vi "find_InstrumentObject_by_Name.vi"(10 "Instrument Name":string, 11 "InstrumentObjects":refnum<class "instrument.lvclass">[](array[class])) -> (0 "found?":bool, 1 "index of found":i32, 2 "found InstrObject out":refnum<class "instrument.lvclass">, 3 "InstrumentObjects out":refnum<class "instrument.lvclass">[](array[class]))   [LabVIEW 2017]
doc: "Find the correct IntrumentObject by the Name of the Instrument"
uses:
  Classes/Instrument/instrument.lvclass
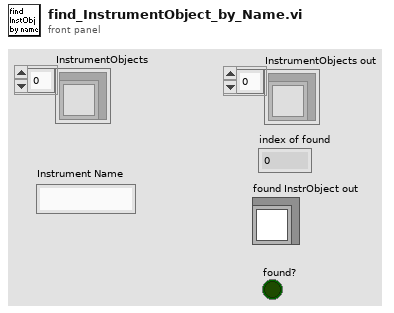
[diagram p1: front panel]
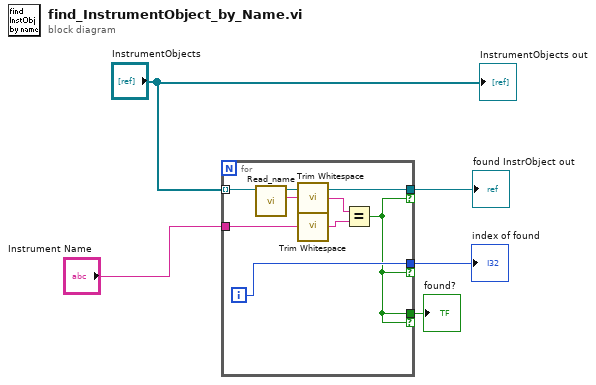
[diagram p0: block diagram]
diagram:
  n1 = for {
    tunnel: "InstrumentObjects" -> [w13] mode=indexing
    tunnel: "Instrument Name" -> [w11]
    tunnel: [w8] -> w4 if=w6
    tunnel: [w7] -> w2 if=w6
    tunnel: [w6] -> w1 if=w6
    i -> [w7]
    n2 = call-dynamic "Read_name.vi"("instrument in"=w13) -> ("name"=w12:string, "instrument out"=w8:refnum<class "instrument.lvclass">)  [unwired: 8 in, 1 out]
    n3 = call <vilib>:"Trim Whitespace.vi"("string"=w12) -> ("trimmed string"=w10:string)  [unwired: 1 in]
    n4 = call <vilib>:"Trim Whitespace.vi"("string"=w11) -> ("trimmed string"=w9:string)  [unwired: 1 in]
    n5 = Equal?(x=w10, y=w9) -> (x = y?=w6:bool)
  }
  "found InstrObject out" <- w4
  "index of found" <- w2
  "found?" <- w1
  "InstrumentObjects out" <- "InstrumentObjects"
